vi "accept connection.vi"(8 "error in":errorcluster, 10 "connection ID":refnum<k5>, 11 "lvlibretls server listener in":refnum<class "lvlibretls server listener.lvclass">) -> (0 "error out":errorcluster, 2 "lvlibretls connection":refnum<class "lvlibretls connection.lvclass">, 3 "lvlibretls server listener out":refnum<class "lvlibretls server listener.lvclass">)   [LabVIEW 2016, in "lvlibretls server listener.lvclass"]
doc: "use an existing server context and a new incoming tcp connection to instantiate a server-oriented tls connection. Technically, I think this could be used to layer a server-side TLS instance over a client side TCP instance, since labview treats both tcp connection types the same."
uses:
  lvlibretls server listener.lvclass
  socket connection/lvlibretls connection.lvclass
  C:/Users/IEUser/Desktop/tlssimple/libretls/context parent/lvlibretls configurable context.lvclass
  context parent/lvlibretls configurable context.lvclass/lvlibretls configurable context.ctl
  lvlibretls server listener.lvclass/lvlibretls server listener.ctl
  context parent/lvlibretls configurable context.lvclass
  lv tls dll.lvlib
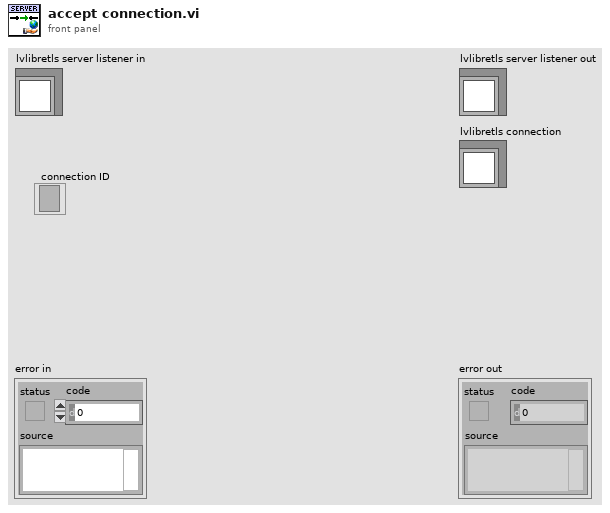
[diagram p1: front panel]
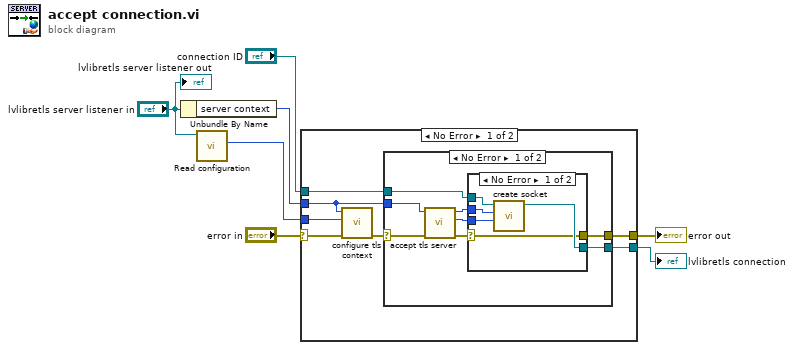
[diagram p0: block diagram]
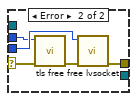
[diagram p2: hidden frame]
diagram:
  n1 = Unbundle By Name("lvlibretls server listener in") -> ("server context"=w1:u64)
  n2 = call "Read configuration.vi"("lvlibretls configurable context in"="lvlibretls server listener in") -> ("configuration"=w5:u64)  [unwired: 10 in]
  n3 = case shown="No Error" "error in" {
    selector: "error in" -> [w11 w34]
    tunnel: [w14 w34] -> w3
    tunnel: "connection ID" -> [w13 _]
    tunnel: [w12 _] -> w6
    tunnel: w5 -> [w10 _]
    tunnel: w1 -> [w9 _]
    frame No Error {
      n4 = call "configure tls context.vi"("error in"=w11, "config"=w10, "context"=w9) -> ("error out"=w8:errorcluster)  [unwired: 8 in]
      n5 = case shown="No Error" w8 {
        selector: w8 -> [w19 w33]
        tunnel: [w16 w33] -> w14
        tunnel: w13 -> [w22 _]
        tunnel: [w20 _] -> w12
        tunnel: w9 -> [w18 _]
        frame No Error {
          n6 = call "accept tls server.vi"("error in"=w19, "client"=w18) -> ("error out"=w17:errorcluster, "lvsocket"=w21:u64, "connection"=w15:u64)  [unwired: 7 in]
          n7 = case shown="No Error" w17 {
            selector: w17 -> [w23 w30]
            tunnel: w22 -> [w27 _]
            tunnel: w21 -> [w26 w31]
            tunnel: [w25 _] -> w20
            tunnel: w15 -> [w24 w28]
            tunnel: [w23 w32] -> w16
            frame No Error {
              n8 = call "create socket.vi"("lvsocket"=w26, "tls socket"=w24, "connection"=w27) -> ("lvlibretls connection out"=w25:refnum<class "lvlibretls connection.lvclass">)  [unwired: 8 in]
            }
            frame Error {
              n9 = call "tls free.vi"("error in"=w30, "tls context"=w28) -> ("error out"=w29:errorcluster)  [unwired: 9 in]
              n10 = call "free lvsocket.vi"("error in"=w29, "lvsocket"=w31) -> ("error out"=w32:errorcluster)  [unwired: 9 in]
            }
          }
        }
        frame Error {
        }
      }
    }
    frame Error {
    }
  }
  "error out" <- w3
  "lvlibretls connection" <- w6
  "lvlibretls server listener out" <- "lvlibretls server listener in"
